vi "Configure.vi"(8 "error in (no error)":errorcluster, 9 "Send Pressure?":bool, 10 "NI_ChannelName":string) -> (0 "error out":errorcluster, 3 "Baratron out":refnum<class "Baratron.lvclass">)   [LabVIEW 2021, in "Baratron.lvclass"]
uses:
  Baratron.lvclass
  Baratron.lvclass/Baratron.ctl
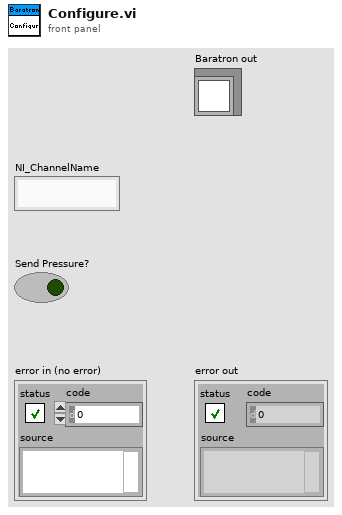
[diagram p1: front panel]
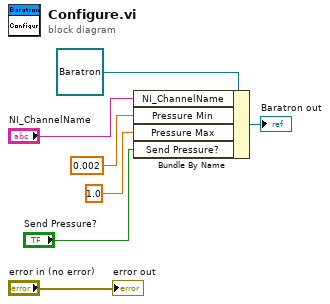
[diagram p0: block diagram]
diagram:
  n1 = Bundle By Name(cluster=refnum<class "Baratron.lvclass"> refnum ("Baratron.lvlib:Baratron.lvclass"), "NI_ChannelName"="NI_ChannelName", "Pressure Min"=0.002, "Pressure Max"=1.0, "Send Pressure?"="Send Pressure?") -> (→"Baratron out":refnum<class "Baratron.lvclass">)
  "error out" <- "error in (no error)"
